vi "Update Current Temperature.vi"(8 "error in (no error)":cluster{"状态":bool, "代码":i32, "源":string} caption="错误输入（无错误）", 10 "当前温度":dbl, 11 "冷却器UI输入":refnum<class "Programmatic Controller.lvclass">) -> (0 "error out":cluster{"状态":bool, "代码":i32, "源":string} caption="错误输出", 3 "冷却器UI输出":refnum<class "Programmatic Controller.lvclass">)   [LabVIEW 2015, in "Programmatic Controller.lvclass"]
doc: "更新记录，写入新的温度报告。"
uses:
  Programmatic Controller.lvclass
  Programmatic Controller.lvclass/Programmatic Controller.ctl
panel:
  in  "新室内温度":string="新室内温度：%f\\n"
  in  "初始室内温度":string="初始室内温度：%f\\n"
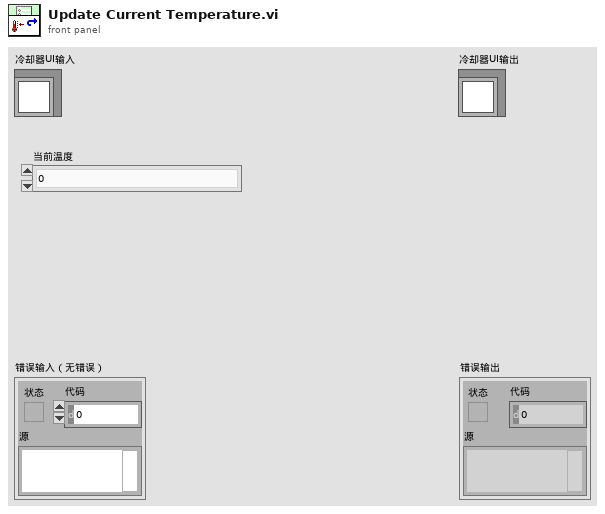
[diagram p1: front panel]
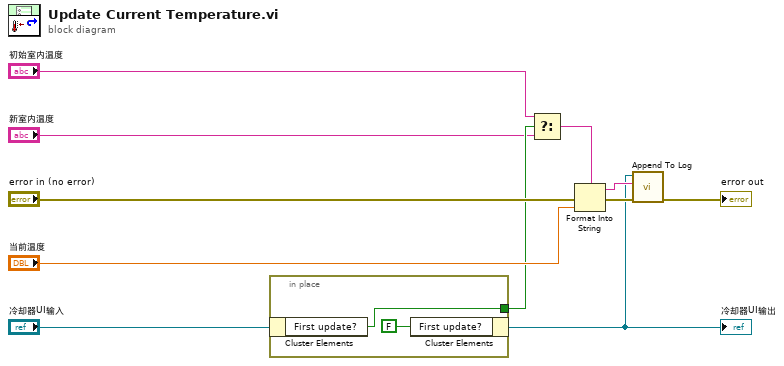
[diagram p0: block diagram]
diagram:
  n1 = in-place {
    in-place-border: [w12] -> w3
    n2 = in-place-cluster #1("冷却器UI输入") -> ("First update?"=w12:bool)
    n3 = in-place-cluster #1("First update?"=FALSE) -> (w4:refnum<class "Programmatic Controller.lvclass">)
  }
  "冷却器UI输出" <- w4
  n4 = Select(t="初始室内温度", s=w3, f="新室内温度") -> (s? t:f=w6:string)
  n5 = Format Into String(format string=w6, error in="error in (no error)", "当前温度") -> (resulting string=w11:string, error out=w10:errorcluster)  [unwired: 1 in]
  n6 = call "Append To Log.vi"("error in (no error)"=w10, "字符串"=w11, "冷却器备用UI输入"=w4) -> ("error out"=→"error out":cluster{"状态":bool, "代码":i32, "源":string})  [unwired: 8 in]
